vi "UI final scorbot.vi"() -> ()   [LabVIEW 2014]
uses:
  <vilib>/userdefined/High Color/IMAQdx.ctl
  <vilib>/myRIO/Instrument Drivers/Onboard IO/DIO/typedefs/DIO Reference.ctl
  <vilib>/myRIO/Common/Instrument Driver Framework/Utilities/typedefs/myRIO Generic Hardware Reference.ctl
  <vilib>/myRIO/Common/Instrument Driver Framework/Utilities/typedefs/Hardware Version Enum.ctl
  <vilib>/myRIO/Common/Instrument Driver Framework/Utilities/typedefs/myRIO v1.0 Reference.ctl
  <vilib>/myRIO/Common/Instrument Driver Framework/Utilities/typedefs/Generic FPGA Reference.ctl
  <vilib>/myRIO/Common/Instrument Driver Framework/myRIO v1.0/DIO/typedefs/DIO Channels List.ctl
  <vilib>/myRIO/Common/Instrument Driver Framework/myRIO v1.0/DIO/typedefs/DIO Channels Enum.ctl
  <vilib>/userdefined/High Color/nirio_resource_hc.ctl
  <vilib>/myRIO/Common/Instrument Driver Framework/Utilities/vis/Is FPGA Ref Available.vi
  <vilib>/myRIO/Common/Instrument Driver Framework/myRIO v1.0/DIO/vis/myRIO v1.1 Open DIO.vi
  <vilib>/myRIO/Instrument Drivers/Onboard IO/DIO/vis/Read.vi
  <vilib>/myRIO/Common/Instrument Driver Framework/Utilities/vis/Validate Channels.vi
  <vilib>/myRIO/Common/Instrument Driver Framework/myRIO v1.0/DIO/vis/myRIO v1.0 Reserve DIO.vi
  <vilib>/myRIO/Common/Instrument Driver Framework/myRIO v1.0/UART/vis/myRIO v1.0 Close UART.vi
  <vilib>/myRIO/Common/Instrument Driver Framework/myRIO v1.0/Resource Manager/vis/myRIO v1.0 Reserve Channel List.vi
  <vilib>/myRIO/Common/Instrument Driver Framework/myRIO v1.0/DIO/vis/myRIO v1.0 Build MUX Configuration DIO.vi
  <vilib>/myRIO/Common/Instrument Driver Framework/myRIO v1.0/Resource Manager/vis/myRIO v1.0 Reserve Channel.vi
  <vilib>/myRIO/Common/Instrument Driver Framework/myRIO v1.0/Resource Manager/vis/myRIO v1.0 Unreserve Channel.vi
  <vilib>/myRIO/Common/Instrument Driver Framework/myRIO v1.0/Resource Manager/vis/myRIO v1.0 Create Configuration List.vi
  <vilib>/myRIO/Common/Instrument Driver Framework/myRIO v1.0/Resource Manager/vis/myRIO v1.0 Build Mutex Name.vi
  <vilib>/Utility/VariantDataType/GetNumericInfo.vi
  <vilib>/Utility/error.llb/Error Cluster From Error Code.vi
  <vilib>/myRIO/Common/Instrument Driver Framework/myRIO v1.0/myRIO v1.1 Open.vi
  <vilib>/myRIO/Common/Instrument Driver Framework/Utilities/vis/IO Manager.vi
  <vilib>/myRIO/Common/Instrument Driver Framework/Utilities/vis/Configuration Manager.vi
  <vilib>/myRIO/Common/Instrument Driver Framework/myRIO v1.0/Resource Manager/vis/myRIO v1.0 Configure IO.vi
  <vilib>/myRIO/Common/Instrument Driver Framework/myRIO v1.0/myRIO v1.0 Close.vi
  <vilib>/myRIO/Common/Instrument Driver Framework/myRIO v1.0/DIO/vis/myRIO v1.0 Read DIO.vi
  <vilib>/addons/control/pid/pid.llb/PID (DBL).vi
  <vilib>/myRIO/Common/Instrument Driver Framework/Utilities/vis/FPGA Ref Manager.vi
  <vilib>/myRIO/Common/Instrument Driver Framework/myRIO v1.0/myRIO v1.0 Reset FPGA.vi
  <vilib>/myRIO/Common/Instrument Driver Framework/myRIO v1.0/IRQ/vis/myRIO v1.0 IRQ Info FGV.vi
  <vilib>/myRIO/Common/Instrument Driver Framework/myRIO v1.0/IRQ/vis/myRIO v1.0 Timer IRQ Info FGV.vi
  <vilib>/myRIO/Common/Instrument Driver Framework/myRIO v1.0/IRQ/vis/myRIO v1.0 ISR Agent.vi
  <vilib>/Utility/inputDevices.llb/joystickAcquire.vi
  <vilib>/myRIO/Express VI/Onboard IO/DI/DI Express VI.xnode
  <vilib>/myRIO/Instrument Drivers/Onboard IO/DIO/vis/myRIO DIO Open.xnode
  <vilib>/myRIO/Instrument Drivers/Onboard IO/DIO/DIO.lvlib
  <vilib>/addons/control/pid/NI_PID_pid.lvlib
  <vilib>/myRIO/Instrument Drivers/Utilities/Utilities.lvlib
  <vilib>/vision/NI_Vision_Development_Module.lvlib
  <vilib>/vision/driver/NI_Vision_Acquisition_Software.lvlib
panel:
  out "output cluster 5":T1
  out "Numeric 3":dbl
  in  "Reset1":bool
  out "device ID":refnum<k1>
  out "dtheta2":i32
  out "dtheta3":i32
  out "dt":u32
  out "error out 2":errorcluster
  out "output cluster 4":cluster{dbl, dbl}
  out "output cluster 3":cluster{dbl, dbl}
  out "output cluster 2":cluster{dbl, dbl}
  in  "stop VI":bool
  in  "Tab Control":enum32{"Control", "Train"}(tab)
  out "B/DIO3 (Pin 17)":bool
  out "B/DIO2 (Pin 15)":bool
  out "B/DIO4 (Pin 19)":bool
  out "B/DIO5 (Pin 21)":bool
  out "B/DIO6 (Pin 23)":bool
  out "B/DIO7 (Pin 25)":bool
  out "Counter Value 1":dbl
  in  "PID gains 2":T2={"proportional gain (Kc)"=-0.5, "integral time (Ti, min)"=0.0, "derivative time (Td, min)"=0.0} {"derivative time (Td, min)" format="%.3f"; "integral time (Ti, min)" format="%.3f"; "proportional gain (Kc)" format="%.3f"}
  in  "PID gains":T2={"proportional gain (Kc)"=-0.1, "integral time (Ti, min)"=0.0, "derivative time (Td, min)"=0.0} {"derivative time (Td, min)" format="%.3f"; "integral time (Ti, min)" format="%.3f"; "proportional gain (Kc)" format="%.3f"}
  out "Omega3":dbl
  out "Omega2":dbl
  out "Elbow angle":dbl
  in  "Max Angle 3":dbl=90.0
  in  "Min angle 3":dbl=-120.0
  in  "Max Encoder Value 3":dbl=-62000.0
  in  "Min Encoder Value 3":dbl
  out "Shoulder angle":dbl
  in  "Max Angle 2":dbl=120.0
  in  "Min angle 2":dbl
  in  "Max Encoder Value 2":dbl=27000.0
  in  "Min Encoder Value 2":dbl
  out "Base angle":dbl
  in  "Max Angle":dbl=90.0
  in  "Min angle":dbl=-90.0
  in  "Max Encoder Value":dbl=-570.0
  in  "Min Encoder Value":dbl
  in  "Reset":bool
  out "Counter Value 3":i32
  out "Counter Value 2":i32
  out "direction info":T3
  out "button info":T4
  out "axis info":T5
  in  "Tab Control 2":enum32{"Learn", "Perform"}(tab)
  in  "Stop counting":bool
  in  "NEXT":bool
  in  "Tab Control 3":enum32{"Normal training", "Train using Vision"}(tab)=enum."Train using Vision"
  out "Encoders initialised":bool
  in  "Save":bool
  out "output cluster":T6
  in  "Save":bool
  in  "Red or Hue Range":cluster{dbl, dbl}(slide)={0.0, 255.0} scale=0.0..255.0
  out "box area":dbl
  in  "Session In":T7="cam0"
  out "object height":i32
  out "object width":i32
  out "Bottom y-displacement":i32
  out "Right x-displacement":i32
  out "Top y-displacement":i32
  out "Left x-displacement":i32
  out "centroid y-displacement":sgl
  out "centroid x-displacement":sgl
  out "threshold":T8(plugin-control)
  in  "Blue or Luma or Val or Inten Range":cluster{dbl, dbl}(slide)={0.0, 255.0} scale=0.0..255.0
  out "Object Info":T9
  out "Largest Area":sgl
  out "Found Objects":T10(array[cluster]) {"Aspect Ratio" format="%.2f"; "Orientation" format="%.2f"; "Area" format="%.2f"; "Object Center"."Y" format="%.2f"; "Object Center"."X" format="%.2f"}
  out "Number of Objects":i32
  out "live feed":T8(plugin-control)
  in  "Green or Sat Range":cluster{dbl, dbl}(slide)={0.0, 255.0} scale=0.0..255.0
  in  "stop vision":bool
  out "Vision initialised":bool
  out "steps":dbl
  out "Set Elbow":dbl
  out "Set Shoulder":dbl
  out "Set Base":dbl
  in  "NeXT step":dbl
  in  "Max Encoder3":dbl=-118000.0
  in  "Max Encoder 2":dbl=27000.0
  out "data out":dbl[][](array[numeric])
  out "Current Angle 1":dbl
  out "Counter1":dbl
  out "B/DIO3 (Pin 17) 2":bool
  out "B/DIO2 (Pin 15) 2":bool
  out "Set Point1":dbl
  out "direction_1b":bool
  out "direction_1a":bool
  in  "Max Encoder1":dbl=-3300.0
  in  "Reset1":bool
  in  "Set Point Angle1":dbl
  in  "Min Encoder1":dbl
  in  "Min Angle1":dbl=-90.0
  in  "Max Angle1":dbl=90.0
  out "error 3":dbl
  in  "Enable1":bool=TRUE
  out "Current Angle3":dbl
  out "direction_3b":bool
  out "B/DIO6 (Pin 23) 2":bool
  out "B/DIO7 (Pin 25) 2":bool
  out "dirction_3a":bool
  out "Set Point3":dbl
  in  "Reset3":bool
  in  "Set Point Angle3":dbl
  out "Numeric3":dbl
  out "Omega3 2":dbl
  out "dt 2":u32
  out "dtheta":i32
  in  "Min Encoder3":dbl
  in  "Min Angle3":dbl=-120.0
  in  "Max Angle3":dbl=90.0
  out "error3":dbl
  out "Counter Value3":i32
  out "B/DIO5 (Pin 21) 2":bool
  out "B/DIO4 (Pin 19) 2":bool
  out "direction 2b":bool
  out "direction 2a":bool
  out "Current Angle2":dbl
  in  "Reset 2":bool
  in  "Set Point Angle2":dbl
  out "Numeric2":dbl
  out "Omega 2":dbl
  out "dt 3":u32
  out "dtheta 2":i32
  in  "PID gains 4":T2={"proportional gain (Kc)"=-0.5, "integral time (Ti, min)"=0.0, "derivative time (Td, min)"=0.0} {"derivative time (Td, min)" format="%.3f"; "integral time (Ti, min)" format="%.3f"; "proportional gain (Kc)" format="%.3f"}
  in  "Min Encoder2":dbl
  in  "Min Angle2":dbl
  in  "Max Angle2":dbl=120.0
  out "error 2":dbl
  in  "Set Point2":dbl
  out "Counter Value2":i32
  in  "PID gains 3":T2={"proportional gain (Kc)"=-0.1, "integral time (Ti, min)"=0.0, "derivative time (Td, min)"=0.0} {"derivative time (Td, min)" format="%.3f"; "integral time (Ti, min)" format="%.3f"; "proportional gain (Kc)" format="%.3f"}
  out "Array":dbl[][](array[numeric])
  out "Array 2":dbl[][](array[numeric])
  out "Array 3":dbl[][](array[numeric])
  out "Array 4":dbl[][](array[numeric])
  out "Array 5":dbl[][](array[numeric])
  out "Array 6":dbl[][](array[numeric])
types:
  T1 = cluster{dbl[][], dbl[][], dbl[][], dbl[][], dbl[][], dbl[][]}
  T2 = cluster{"proportional gain (Kc)":dbl, "integral time (Ti, min)":dbl, "derivative time (Td, min)":dbl}
  T3 = cluster{"pov 1":i32, "pov 2":i32, "pov 3":i32, "pov 4":i32}
  T4 = cluster{"button 1":bool, "button 2":bool, "button 3":bool, "button 4":bool, "button 5":bool, "button 6":bool, "button 7":bool, "button 8":bool, "button 9":bool, "button 10":bool, "button 11":bool, "button 12":bool, "button 13":bool, "button 14":bool, "button 15":bool, "button 16":bool, "button 17":bool, "button 18":bool, "button 19":bool, "button 20":bool, "button 21":bool, "button 22":bool, "button 23":bool, "button 24":bool, "button 25":bool, "button 26":bool, "button 27":bool, "button 28":bool, "button 29":bool, "button 30":bool, "button 31":bool, "button 32":bool}
  T5 = cluster{"X axis":i32, "Y axis":i32, "Z axis":i32, "X axis rotation":i32, "Y axis rotation":i32, "Z axis rotation":i32, "U axis":i32, "V axis":i32}
  T6 = cluster{"Elbow angle":dbl, "Base angle":dbl, "Shoulder angle":dbl}
  T7 = typedef "IMAQdx.ctl" = refnum<k21>
  T8 = typedef "IMAQ Image.ctl" = refnum<image>
  T9 = cluster{"Object Center":cluster{"X":sgl, "Y":sgl}, "Bounding Box":cluster{"X Left":i32, "Y Top":i32, "X Right":i32, "Y Bottom":i32}, "Area":sgl, "Orientation":sgl, "Aspect Ratio":sgl, "Nb Holes":i32}
  T10 = cluster{"Object Center":cluster{"X":sgl, "Y":sgl}, "Bounding Box":cluster{"X Left":i32, "Y Top":i32, "X Right":i32, "Y Bottom":i32}, "Area":sgl, "Orientation":sgl, "Aspect Ratio":sgl, "Nb Holes":i32}[]
  T11 = cluster{"Objects":u16, "Threshold":i32, "Reject Border":bool, "Fill Holes":bool, "Min Object Size":bool, "Min Size":i32, "Max Object Size":bool, "Max Size":i32, "Show Search Area":bool, "Show Center":bool, "Show Bounding Box":bool}
  T12 = typedef "DIO.lvlib/DIO Reference.ctl" = cluster{"myRIO Reference":T13, "DIO Channels List":T17}
  T13 = typedef "myRIO Generic Hardware Reference.ctl" = cluster{"myRIO Model":T14, "myRIO Hardware Reference":T15}
  T14 = typedef "Hardware Version Enum.ctl" = enum16{"Unknown", "myRIO-1900", "myRIO-1950"}
  T15 = typedef "myRIO v1.0 Reference.ctl" = cluster{"Generic FPGA Reference":T16, "Allow multiple opens":bool}
  T16 = typedef "Generic FPGA Reference.ctl" = refnum<k20>
  T17 = typedef "DIO Channels List.ctl" = T18[]
  T18 = typedef "DIO Channels Enum.ctl" = enum16{"Not Connected", "C/DIO0", "C/DIO1", "C/DIO2", "C/DIO3", "C/DIO4", "C/DIO5", "C/DIO6", "C/DIO7", "A/DIO0", "A/DIO1", "A/DIO2", "A/DIO3", "A/DIO4", "A/DIO5", "A/DIO6", "A/DIO7", "A/DIO8", "A/DIO9", "A/DIO10", "A/DIO11", "A/DIO12", "A/DIO13", "A/DIO14", "A/DIO15", "B/DIO0", "B/DIO1", "B/DIO2", "B/DIO3", "B/DIO4", "B/DIO5", "B/DIO6", "B/DIO7", "B/DIO8", "B/DIO9", "B/DIO10", "B/DIO11", "B/DIO12", "B/DIO13", "B/DIO14", "B/DIO15", "LED0", "LED1", "LED2", "LED3", "Button0"}
  T19 = typedef "nirio_resource_hc.ctl" = tag
  T20 = typedef "Image Type" = u32
  T21 = cluster{"X Left":i32, "Y Top":i32, "X Right":i32, "Y Bottom":i32}
  T22 = typedef "NI_Matrix.lvlib/RealMatrix.ctl" = dbl[][]
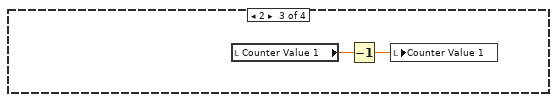
[diagram p8: hidden frame]
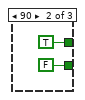
[diagram p10: hidden frame]
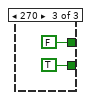
[diagram p11: hidden frame]
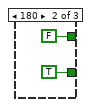
[diagram p12: hidden frame]
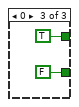
[diagram p13: hidden frame]
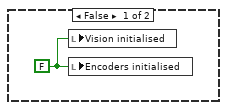
[diagram p16: hidden frame]
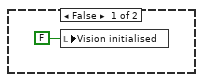
[diagram p17: hidden frame]
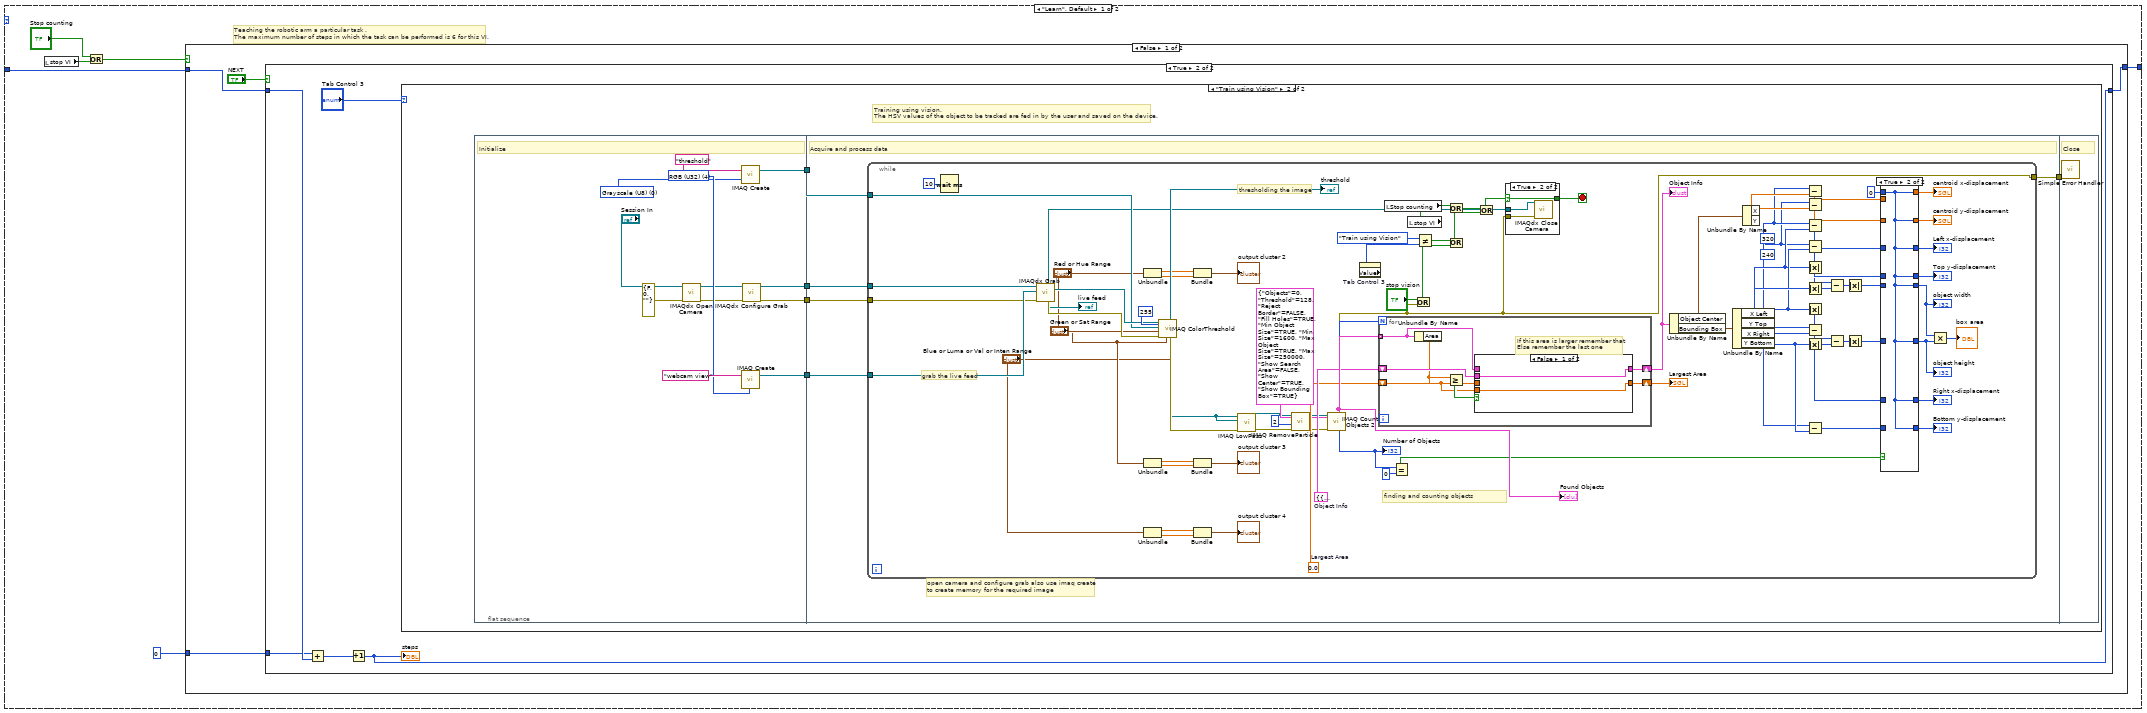
[diagram p19: hidden frame]
diagram:
  # "You can configure the Accelerometer Express VI by double-clicking it.\nYou can find other myRIO Express VIs in the myRIO palette."
  n1 = flat-sequence {
    tunnel: [errorcluster {"status"=FALSE, "code"=0, "source"=""} ("error out")] -> w3
    tunnel: [w4] -> w2
    tunnel: w3 -> [w9]
    tunnel: w2 -> [w10]
    tunnel: [w6] -> w1
    tunnel: w1 -> [w799]
    frame #0 {
      # "train1"
      # "#CodeNeeded - Add code to initialize your user interface and hardware here."
      # "Initialize"
      n2 = call <vilib>:"Initialize Joystick.vi"() -> ("device ID"=w4:refnum<k1>)  [unwired: 10 in, 1 out]
      "device ID" <- w4
    }
    frame #1 {
      # "Network Stream:\nFile Reader and Writer"
      # "train1"
      # "n3"
      # "n2"
      # "n1"
      # "host VI"
      # "Acquire and process data"
      n3 = while {
        shift-right: [w137] -> _
        shift-left: _ -> [w136]
        tunnel: w10 -> [w121]
        stop <- "stop VI" stop-if-true
        # "Network streams are used to transfer the encoder and \nvision data from myRio to the computer and vice versa."
        # "n3"
        # "n2"
        # "n1"
        n4 = local read "Tab Control 2"() -> (w134:enum32{"Learn", "Perform"})
        n5 = local read "Tab Control"() -> (w132:enum32{"Control", "Train"})
        n6 = case shown="\"Train\"" "Tab Control" {
          tunnel: [w149 w152] -> w137
          tunnel: w136 -> [w149 w151]
          tunnel: w121 -> [_ _]
          frame "Control", Default {
          }
          frame "Train" {
            # "Training the robotic arm by moving it using joystick.\nThe initial and final encoder readings of each arm are \nbeing transferred to the computer in each step."
            n7 = case shown="\"Perform\"" "Tab Control 2" {
              tunnel: [w158 w302] -> w152
              tunnel: w151 -> [w156 w302]
              frame "Learn", Default {
                # "Teaching the robotic arm a particular task .\nThe maximum number of steps in which the task can be performed is 6 for this VI."
                n8 = local read "stop VI"() -> (w154:bool)
                n9 = Or(x="Stop counting", y=w154) -> (x .or. y?=w153:bool)
                n10 = case shown="False" w153 {
                  tunnel: [w162 w301] -> w158
                  tunnel: 0 -> [w160 w299]
                  tunnel: w156 -> [w159 w300]
                  frame False {
                    n11 = case shown="True" "NEXT" {
                      tunnel: [w163 w165] -> w162
                      tunnel: w159 -> [w163 w167]
                      tunnel: w160 -> [_ w166]
                      frame False {
                      }
                      frame True {
                        n12 = Add(x=w166, y=w167) -> (x+y=w168:i32)
                        n13 = Increment(x=w168) -> (x+1=w165:i32)
                        "steps" <- w165
                        n14 = case shown="\"Train using Vision\"" "Tab Control 3" {
                          frame "Normal training", Default {
                            # "Training by storing encoder readings"
                          }
                          frame "Train using Vision" {
                            # "Training using vision. \nThe HSV values of the object to be tracked are fed in by the user and saved on the device."
                            n15 = flat-sequence {
                              tunnel: [w183] -> w173
                              tunnel: [w180] -> w172
                              tunnel: [w177] -> w171
                              tunnel: [w174] -> w170
                              tunnel: w173 -> [w189]
                              tunnel: [w186] -> w169
                              tunnel: w172 -> [w188]
                              tunnel: w171 -> [w187]
                              tunnel: w170 -> [w190]
                              tunnel: w169 -> [w298]
                              frame #0 {
                                w175 = T20 0 items=["Grayscale (U8)", "Grayscale (I16)", "Grayscale (SGL)", "Complex (CSG)", "RGB (U32)", "HSL (U32)", "RGB (U64)", "Grayscale (U16)"] ("Image Type")
                                w184 = T20 4 items=["Grayscale (U8)", "Grayscale (I16)", "Grayscale (SGL)", "Complex (CSG)", "RGB (U32)", "HSL (U32)", "RGB (U64)", "Grayscale (U16)"] ("Image Type")
                                # "Initialize"
                                n16 = call <vilib>:"IMAQdx Open Camera.vi"("error in"=errorcluster {"status"=FALSE, "code"=0, "source"=""} ("error out"), "Session In"="Session In") -> ("error out"=w179:errorcluster, "Session Out"=w181:T7)  [unwired: 8 in]
                                n17 = call "IMAQ Create"("Image Name"="threshold", "Image Type"=w175) -> ("New Image"=w174:T8)  [unwired: 3 in, 1 out]
                                n18 = call "IMAQ Create"("Image Name"="webcam view", "Image Type"=w184) -> ("New Image"=w183:T8)  [unwired: 3 in, 1 out]
                                n19 = call <vilib>:"IMAQdx Configure Grab.vi"("error in"=w179, "Session In"=w181) -> ("error out"=w177:errorcluster, "Session Out"=w180:T7)  [unwired: 8 in]
                              }
                              frame #1 {
                                # "open camera and configure grab also use imaq create \nto create memory for the required image"
                                # "Acquire and process data"
                                n20 = while {
                                tunnel: w190 -> [w225]
                                tunnel: w189 -> [w224]
                                tunnel: w188 -> [w215]
                                tunnel: w187 -> [w223]
                                tunnel: [w213] -> w186
                                stop <- w216 stop-if-true
                                w230 = 240
                                w232 = 320
                                w269 = T9 {"Object Center"={"X"=0.0, "Y"=0.0}, "Bounding Box"={"X Left"=0, "Y Top"=0, "X Right"=0, "Y Bottom"=0}, "Area"=0.0, "Orientation"=0.0, "Aspect Ratio"=0.0, "Nb Holes"=0}  # Object Info
                                w268 = sgl 0.0  # Largest Area
                                # "finding and counting objects"
                                # "thresholding the image"
                                # "grab the live feed"
                                n21 = Wait (ms)(milliseconds to wait=u32 10) -> ()  [unwired: 1 out]
                                n22 = call <vilib>:"IMAQdx Grab.vi"("error in"=w223, "Image In"=w224, "Session In"=w215) -> ("error out"=w273:errorcluster, "Image Out"=w271:T8, "Session Out"=w214:T7)  [unwired: 5 in, 1 out]
                                "live feed" <- w271
                                n23 = Unbundle("Red or Hue Range") -> (w199:dbl, w198:dbl)
                                n24 = Unbundle("Green or Sat Range") -> (w197:dbl, w196:dbl)
                                n25 = Unbundle("Blue or Luma or Val or Inten Range") -> (w195:dbl, w194:dbl)
                                n26 = call "IMAQ ColorThreshold"("Blue or Luma or Val or Inten Range"="Blue or Luma or Val or Inten Range", "Replace Value"=255, "Green or Sat Range"="Green or Sat Range", "error in (no error)"=w273, "Red or Hue Range"="Red or Hue Range", "Image Dst"=w225, "Image Src"=w271) -> ("error out"=w266:errorcluster, "Image Dst Out"=w265:T8)  [unwired: 3 in]
                                "threshold" <- w265
                                n27 = Bundle(w199, w198) -> (→"output cluster 2":cluster{dbl, dbl})  [unwired: 1 in]
                                n28 = Bundle(w197, w196) -> (→"output cluster 3":cluster{dbl, dbl})  [unwired: 1 in]
                                n29 = Bundle(w195, w194) -> (→"output cluster 4":cluster{dbl, dbl})  [unwired: 1 in]
                                n30 = call "IMAQ LowPass"("Image Src"=w265, "Image Mask"=w265, "error in (no error)"=w266) -> ("Image Dst Out"=w227:T8, "error out"=w229:errorcluster)  [unwired: 4 in]
                                n31 = call "IMAQ RemoveParticle"("error in (no error)"=w229, "Number of Erosion"=2, "Image Src"=w227) -> ("error out"=w228:errorcluster, "Image Dst Out"=w226:T8)  [unwired: 7 in]
                                n32 = call "IMAQ Count Objects 2"("Settings"=T11 {"Objects"=0, "Threshold"=128, "Reject Border"=FALSE, "Fill Holes"=TRUE, "Min Object Size"=TRUE, "Min Size"=1600, "Max Object Size"=TRUE, "Max Size"=250000, "Show Search Area"=FALSE, "Show Center"=TRUE, "Show Bounding Box"=TRUE}, "error in (no error)"=w228, "Image"=w226) -> ("error out"=w213:errorcluster, "Number of Objects"=w259:i32, "Objects"=w270:T10)  [unwired: 4 in, 2 out]
                                "Number of Objects" <- w259
                                "Found Objects" <- w270
                                n33 = property on="Tab Control 3" class="TabCtl (strict)"() -> ("Value"=w210:enum32{"Normal training", "Train using Vision"})  [unwired: 2 in, 2 out]
                                n34 = for {
                                N: w259 -> [_]
                                tunnel: w270 -> [w290] mode=indexing
                                shift-right: [w293] -> w267
                                shift-left: w268 -> [w287]
                                shift-right: [w292] -> w264
                                shift-left: w269 -> [w291]
                                # "If this area is larger remember that\nElse remember the last one"
                                n35 = Unbundle By Name(w290) -> ("Area"=w289:sgl)
                                n36 = Greater Or Equal?(x=w289, y=w287) -> (x >= y?=w288:bool)
                                n37 = case shown="False" w288 {
                                tunnel: [w295 w297] -> w293
                                tunnel: w289 -> [_ w297]
                                tunnel: w287 -> [w295 _]
                                tunnel: [w294 w296] -> w292
                                tunnel: w291 -> [w294 _]
                                tunnel: w290 -> [_ w296]
                                frame False {
                                }
                                frame True {
                                }
                                }
                                }
                                "Largest Area" <- w267
                                "Object Info" <- w264
                                n38 = local read "Stop counting"() -> (w207:bool)
                                n39 = Equal?(x=w259, y=0) -> (x = y?=w257:bool)
                                n40 = local read "stop VI"() -> (w206:bool)
                                n41 = Or(x="stop vision", y=w213) -> (x .or. y?=w211:bool)
                                n42 = Not Equal?(x=enum32{"Normal training", "Train using Vision"}."Train using Vision" ("Tab Control 3"), y=w210) -> (x != y?=w212:bool)
                                n43 = Or(x=w207, y=w206) -> (x .or. y?=w205:bool)
                                n44 = Or(x=w212, y=w211) -> (x .or. y?=w204:bool)
                                n45 = Or(x=w205, y=w204) -> (x .or. y?=w203:bool)
                                n46 = case shown="True" w203 {
                                selector: w203 -> [_ w276]
                                tunnel: w213 -> [_ w275]
                                tunnel: [FALSE w276] -> w216
                                tunnel: w214 -> [_ w277]
                                frame False {
                                }
                                frame True {
                                n47 = call <vilib>:"IMAQdx Close Camera.vi"("error in"=w275, "Session In"=w277) -> ()  [unwired: 9 in, 1 out]
                                }
                                }
                                n48 = Unbundle By Name(w264) -> ("Object Center"=w263:cluster{"X":sgl, "Y":sgl}, "Bounding Box"=w261:T21)
                                n49 = Unbundle By Name(w261) -> ("X Left"=w233:i32, "Y Top"=w234:i32, "X Right"=w235:i32, "Y Bottom"=w231:i32)
                                n50 = Unbundle By Name(w263) -> ("X"=w237:sgl, "Y"=w236:sgl)
                                n51 = Subtract(x=w232, y=w237) -> (x-y=w251:sgl)
                                n52 = Subtract(x=w230, y=w236) -> (x-y=w250:sgl)
                                n53 = Subtract(x=w232, y=w233) -> (x-y=w249:i32)
                                n54 = Subtract(x=w230, y=w234) -> (x-y=w248:i32)
                                n55 = Absolute Value(x=w233) -> (abs(x)=w243:i32)
                                n56 = Absolute Value(x=w235) -> (abs(x)=w242:i32)
                                n57 = Absolute Value(x=w234) -> (abs(x)=w245:i32)
                                n58 = Subtract(x=w232, y=w235) -> (x-y=w247:i32)
                                n59 = Absolute Value(x=w231) -> (abs(x)=w244:i32)
                                n60 = Subtract(x=w230, y=w231) -> (x-y=w246:i32)
                                n61 = Subtract(x=w243, y=w242) -> (x-y=w241:i32)
                                n62 = Subtract(x=w245, y=w244) -> (x-y=w239:i32)
                                n63 = Absolute Value(x=w241) -> (abs(x)=w240:i32)
                                n64 = Absolute Value(x=w239) -> (abs(x)=w238:i32)
                                n65 = case shown="True" w257 {
                                tunnel: [w285 w286] -> w222
                                tunnel: 0 -> [_ w286]
                                tunnel: [w284 w286] -> w221
                                tunnel: [w283 w286] -> w255
                                tunnel: [w281 w286] -> w254
                                tunnel: [w282 w286] -> w253
                                tunnel: [w280 w286] -> w252
                                tunnel: w251 -> [w285 _]
                                tunnel: w250 -> [w284 _]
                                tunnel: w249 -> [w283 _]
                                tunnel: w248 -> [w282 _]
                                tunnel: w247 -> [w281 _]
                                tunnel: w246 -> [w280 _]
                                tunnel: [w279 w286] -> w219
                                tunnel: w240 -> [w279 _]
                                tunnel: [w278 w286] -> w218
                                tunnel: w238 -> [w278 _]
                                frame False {
                                }
                                frame True {
                                }
                                }
                                "centroid x-displacement" <- w222
                                "centroid y-displacement" <- w221
                                "Left x-displacement" <- w255
                                "Top y-displacement" <- w253
                                "Right x-displacement" <- w254
                                "Bottom y-displacement" <- w252
                                "object width" <- w219
                                "object height" <- w218
                                n66 = Multiply(x=w219, y=w218) -> (x*y=→"box area":i32)
                                }
                              }
                              frame #2 {
                                # "Close"
                                n67 = call <vilib>:"Simple Error Handler.vi"("error in (no error)"=w298) -> ()  [unwired: 4 in, 5 out]
                              }
                            }
                          }
                        }
                      }
                    }
                  }
                  frame True {
                    n68 = Multiply(x=w299, y=w300) -> (x*y=w301:i32)
                  }
                }
              }
              frame "Perform" {
                # "The Robotic arm performs the task autonomously in steps.\nThe myRio reads the initial and final encoder readings from the file on \ncomputer and actuates the motors accordingly to reach the desired position."
                n69 = while {
                  tunnel: [w366] -> _
                  shift-right: [w482] -> _
                  shift-left: _ -> [w483]
                  shift-right: [w479] -> _
                  shift-left: _ -> [w481]
                  shift-right: [w478] -> _
                  shift-left: _ -> [w480]
                  shift-right: [w421] -> _
                  shift-left: _ -> [w424]
                  shift-right: [w420] -> _
                  shift-left: _ -> [w423]
                  shift-right: [w419] -> _
                  shift-left: _ -> [w422]
                  shift-right: [w364] -> _
                  shift-left: _ -> [w365]
                  stop <- w304 stop-if-true
                  # "PID for speed control"
                  # "PID for speed control"
                  n70 = local read "output cluster 5"() -> (w315:T1)
                  n71 = local read "Tab Control 2"() -> (w307:enum32{"Learn", "Perform"})
                  n72 = local read "Set Shoulder"() -> (w310:dbl)
                  n73 = local read "Set Point1"() -> (w346:dbl)
                  n74 = local read "Set Elbow"() -> (w309:dbl)
                  n75 = local read "Counter1"() -> (w336:dbl)
                  n76 = local read "Set Base"() -> (w308:dbl)
                  n77 = local write "Set Point Angle2"(w310) -> ()
                  n78 = local write "Set Point Angle1"(w308) -> ()
                  n79 = case shown="True" "Reset1" {
                    frame False {
                    }
                    frame True {
                      n80 = local write "Counter1"(0.0 ("Counter")) -> ()
                    }
                  }
                  n81 = local write "Set Point Angle3"(w309) -> ()
                  n82 = case shown="0, Default" "NeXT step" {
                    tunnel: w315 -> [_ w492 w505 w514 w523 w531 w541]
                    tunnel: [w491 w499 w503 w512 w521 w530 w539] -> w313
                    tunnel: [w490 w495 w502 w511 w520 w529 w538] -> w312
                    tunnel: [w489 w494 w501 w510 w519 w528 w537] -> w311
                    frame 0, Default {
                      n83 = local read "Current Angle 1"() -> (w490:dbl)
                      n84 = local read "Current Angle3"() -> (w491:dbl)
                      n85 = local read "Current Angle2"() -> (w489:dbl)
                    }
                    frame 1 {
                      w496 = 0 ("index (col)")
                      n86 = Unbundle(w492) -> (w493:dbl[][])  [unwired: 5 out]
                      n87 = Index Array(array=w493, index (row) #1=0 ("index (row)"), index (col) #1=w496, index (row) #2=1 ("index (row)"), index (col) #2=w496, index (row) #3=2 ("index (row)"), index (col) #3=w496) -> (element #1=w499:dbl, element #2=w495:dbl, element #3=w494:dbl)
                    }
                    frame 2 {
                      w506 = 0 ("index (col)")
                      n88 = Unbundle(w505) -> (w504:dbl[][])  [unwired: 5 out]
                      n89 = Index Array(array=w504, index (row) #1=0 ("index (row)"), index (col) #1=w506, index (row) #2=1 ("index (row)"), index (col) #2=w506, index (row) #3=2 ("index (row)"), index (col) #3=w506) -> (element #1=w503:dbl, element #2=w502:dbl, element #3=w501:dbl)
                    }
                    frame 3 {
                      w515 = 0 ("index (col)")
                      n90 = Unbundle(w514) -> (w513:dbl[][])  [unwired: 5 out]
                      n91 = Index Array(array=w513, index (row) #1=0 ("index (row)"), index (col) #1=w515, index (row) #2=1 ("index (row)"), index (col) #2=w515, index (row) #3=2 ("index (row)"), index (col) #3=w515) -> (element #1=w512:dbl, element #2=w511:dbl, element #3=w510:dbl)
                    }
                    frame 4 {
                      w524 = 0 ("index (col)")
                      n92 = Unbundle(w523) -> (w522:dbl[][])  [unwired: 5 out]
                      n93 = Index Array(array=w522, index (row) #1=0 ("index (row)"), index (col) #1=w524, index (row) #2=1 ("index (row)"), index (col) #2=w524, index (row) #3=2 ("index (row)"), index (col) #3=w524) -> (element #1=w521:dbl, element #2=w520:dbl, element #3=w519:dbl)
                    }
                    frame 5 {
                      w536 = 0 ("index (col)")
                      n94 = Unbundle(w531) -> (w532:dbl[][])  [unwired: 5 out]
                      n95 = Index Array(array=w532, index (row) #1=0 ("index (row)"), index (col) #1=w536, index (row) #2=1 ("index (row)"), index (col) #2=w536, index (row) #3=2 ("index (row)"), index (col) #3=w536) -> (element #1=w530:dbl, element #2=w529:dbl, element #3=w528:dbl)
                    }
                    frame 6 {
                      w542 = 0 ("index (col)")
                      n96 = Unbundle(w541) -> (w540:dbl[][])  [unwired: 5 out]
                      n97 = Index Array(array=w540, index (row) #1=0 ("index (row)"), index (col) #1=w542, index (row) #2=1 ("index (row)"), index (col) #2=w542, index (row) #3=2 ("index (row)"), index (col) #3=w542) -> (element #1=w539:dbl, element #2=w538:dbl, element #3=w537:dbl)
                    }
                  }
                  "Set Elbow" <- w313
                  "Set Base" <- w312
                  "Set Shoulder" <- w311
                  n98 = Not Equal?(x=w307, y=enum32{"Learn", "Perform"}."Perform" ("Tab Control 2")) -> (x != y?=w305:bool)
                  n99 = local read "Numeric 3"() -> (w358:dbl)
                  n100 = local read "Numeric 3"() -> (w356:dbl)
                  n101 = Subtract(x=w336, y=w346) -> (x-y=w361:dbl)
                  "error 3" <- w361
                  n102 = Subtract(x="Max Angle1", y="Min Angle1") -> (x-y=w322:dbl)
                  n103 = Subtract(x="Max Encoder1", y="Min Encoder1") -> (x-y=w321:dbl)
                  n104 = local read "stop VI"() -> (w303:bool)
                  n105 = Subtract(x="Set Point Angle1", y="Min Angle1") -> (x-y=w350:dbl)
                  n106 = Divide(x=w321, y=w322) -> (x/y=w349:dbl)
                  n107 = Divide(x=w322, y=w321) -> (x/y=w320:dbl)
                  n108 = Add(x=1.0 ("upper limit"), y=w358) -> (x+y=w359:dbl)
                  n109 = Subtract(x=-1.0 ("lower limit"), y=w356) -> (x-y=w355:dbl)
                  n110 = xnode "Digital input (1 sample) 7"() -> ("B/DIO6 (Pin 23)"=w384:bool)  [unwired: 1 in, 1 out]
                  "B/DIO6 (Pin 23) 2" <- w384
                  n111 = Or(x=w305, y=w303) -> (x .or. y?=w304:bool)
                  n112 = Multiply(x=w350, y=w349) -> (x*y=w348:dbl)
                  n113 = local read "Counter1"() -> (w319:dbl)
                  n114 = In Range and Coerce(upper limit=w359, x=w361, lower limit=w355) -> (In Range?=w345:bool)  [unwired: 1 out]
                  n115 = Sign(1:w361) -> (0:w363:dbl)
                  n116 = xnode "Digital input (1 sample) 8"() -> ("B/DIO7 (Pin 25)"=w382:bool)  [unwired: 1 in, 1 out]
                  "B/DIO7 (Pin 25) 2" <- w382
                  n117 = case shown="True" w345 {
                    frame False {
                      n118 = local write "Numeric 3"(0.0) -> ()
                    }
                    frame True {
                      n119 = local write "Numeric 3"(0.0) -> ()
                    }
                  }
                  n120 = case shown="1" w363 {
                    tunnel: [TRUE TRUE FALSE] -> w342
                    tunnel: [TRUE FALSE TRUE] -> w343
                    frame 0, Default {
                    }
                    frame 1 {
                    }
                    frame -1 {
                    }
                  }
                  n121 = Add(x=w348, y="Min Encoder1") -> (x+y=w340:dbl)
                  n122 = Multiply(x=w320, y=w319) -> (x*y=w318:dbl)
                  n123 = local write "Set Point1"(w340) -> ()
                  n124 = Add(x="Min Angle1", y=w318) -> (x+y=→"Current Angle 1":dbl)
                  n125 = feedback #1() -> (w385:bool)  [unwired: 1 in]
                  n126 = Not(x=w384) -> (.not. x?=w387:bool)
                  n127 = And(x=w385, y=w382) -> (x .and. y?=w383:bool)
                  "dirction_3a" <- w383
                  n128 = Not(x=w345) -> (.not. x?=w344:bool)
                  n129 = Or(x=w387, y="Reset3") -> (x .or. y?=w394:bool)
                  n130 = And(x=w344, y=w342) -> (x .and. y?=w335:bool)
                  n131 = And(x=w344, y=w343) -> (x .and. y?=w334:bool)
                  n132 = xnode "Digital input (1 sample) 9"() -> ("B/DIO4 (Pin 19)"=w431:bool)  [unwired: 1 in, 1 out]
                  "B/DIO4 (Pin 19) 2" <- w431
                  n133 = case shown="True" "Enable1" {
                    tunnel: w335 -> [_ w627]
                    tunnel: w334 -> [_ w626]
                    tunnel: [FALSE w627] -> w333
                    tunnel: [FALSE w626] -> w323
                    frame False {
                    }
                    frame True {
                    }
                  }
                  n134 = local read "Set Point3"() -> (w395:dbl)
                  n135 = feedback #2() -> (w368:dbl)  [unwired: 1 in]
                  n136 = Subtract(x="Max Encoder3", y="Min Encoder3") -> (x-y=w377:dbl)
                  n137 = Subtract(x="Max Angle3", y="Min Angle3") -> (x-y=w378:dbl)
                  n138 = Tick Count (ms)() -> (millisecond timer value=w419:u32)
                  n139 = xnode "Digital input (1 sample) 12"() -> ("B/DIO2 (Pin 15)"=w337:bool)  [unwired: 1 in, 1 out]
                  "B/DIO2 (Pin 15) 2" <- w337
                  n140 = Divide(x=w378, y=w377) -> (x/y=w373:dbl)
                  n141 = Divide(x=w377, y=w378) -> (x/y=w398:dbl)
                  n142 = Subtract(x="Set Point Angle3", y="Min Angle3") -> (x-y=w399:dbl)
                  n143 = local read "Numeric3"() -> (w406:dbl)
                  n144 = local read "Numeric3"() -> (w404:dbl)
                  n145 = Not(x=w431) -> (.not. x?=w432:bool)
                  n146 = Subtract(x=w419, y=w422) -> (x-y=w410:u32)
                  "dt 2" <- w410
                  n147 = feedback #3() -> (w448:bool)  [unwired: 1 in]
                  n148 = Multiply(x=w399, y=w398) -> (x*y=w397:dbl)
                  n149 = And(x=w448, y=w431) -> (x .and. y?=w427:bool)
                  "direction 2a" <- w427
                  n150 = Add(x=50.0 ("upper limit"), y=w406) -> (x+y=w407:dbl)
                  n151 = Subtract(x=-50.0 ("lower limit"), y=w404) -> (x-y=w403:dbl)
                  n152 = Or(x=w432, y="Reset 2") -> (x .or. y?=w434:bool)
                  n153 = Add(x=w397, y="Min Encoder3") -> (x+y=w396:dbl)
                  n154 = And(x=w333, y=w337) -> (x .and. y?=w324:bool)
                  "direction_1a" <- w324
                  n155 = local write "Set Point3"(w396) -> ()
                  n156 = Subtract(x="Max Encoder 2", y="Min Encoder2") -> (x-y=w446:dbl)
                  n157 = Subtract(x="Max Angle2", y="Min Angle2") -> (x-y=w447:dbl)
                  n158 = xnode "Digital input (1 sample) 11"() -> ("B/DIO3 (Pin 17)"=w330:bool)  [unwired: 1 in, 1 out]
                  "B/DIO3 (Pin 17) 2" <- w330
                  n159 = local read "Set Point2"() -> (w442:dbl)
                  n160 = Divide(x=w446, y=w447) -> (x/y=w438:dbl)
                  n161 = Divide(x=w447, y=w446) -> (x/y=w445:dbl)
                  n162 = Subtract(x="Set Point Angle2", y="Min Angle2") -> (x-y=w439:dbl)
                  n163 = Boolean To (0,1)(Boolean=w324) -> (0, 1=w329:i16)
                  n164 = Tick Count (ms)() -> (millisecond timer value=w478:u32)
                  n165 = Multiply(x=w439, y=w438) -> (x*y=w437:dbl)
                  n166 = local read "Numeric2"() -> (w454:dbl)
                  n167 = local read "Numeric2"() -> (w452:dbl)
                  n168 = Boolean To (0,1)(Boolean=w323) -> (0, 1=w326:i16)
                  n169 = Subtract(x=w478, y=w480) -> (x-y=w460:u32)
                  "dt 3" <- w460
                  n170 = Multiply(x=i16 2, y=w329) -> (x*y=w327:i16)
                  n171 = Add(x=w327, y=w326) -> (x+y=w325:i16)
                  n172 = Add(x=w437, y="Min Encoder2") -> (x+y=w435:dbl)
                  n173 = And(x=w330, y=w323) -> (x .and. y?=w331:bool)
                  "direction_1b" <- w331
                  n174 = Not(x=w330) -> (.not. x?=w341:bool)
                  n175 = Add(x=50.0 ("upper limit"), y=w454) -> (x+y=w455:dbl)
                  n176 = Subtract(x=-50.0 ("lower limit"), y=w452) -> (x-y=w451:dbl)
                  n177 = case shown="1" w325 {
                    frame 0, Default {
                    }
                    frame 1 {
                      n178 = local read "Counter1"() -> (w547:dbl)
                      n179 = Increment(x=w547) -> (x+1=w546:dbl)
                      n180 = local write "Counter1"(w546) -> ()
                    }
                    frame 2 {
                      n181 = local read "Counter1"() -> (w549:dbl)
                      n182 = Decrement(x=w549) -> (x-1=w548:dbl)
                      n183 = local write "Counter1"(w548) -> ()
                    }
                    frame 3 {
                    }
                  }
                  n184 = local write "Set Point2"(w435) -> ()
                  n185 = Or(x=w341, y="Reset1") -> (x .or. y?=w332:bool)
                  n186 = feedback #4() -> (w433:dbl)  [unwired: 1 in]
                  n187 = case shown="True" w332 {
                    frame False {
                    }
                    frame True {
                      n188 = local write "Counter1"(0.0 ("Counter")) -> ()
                    }
                  }
                  n189 = xnode "Digital input (1 sample) 10"() -> ("B/DIO5 (Pin 21)"=w429:bool)  [unwired: 1 in, 1 out]
                  "B/DIO5 (Pin 21) 2" <- w429
                  n190 = feedback #5() -> (w474:bool)  [unwired: 1 in]
                  n191 = feedback #6() -> (w473:bool)  [unwired: 1 in]
                  n192 = case shown="True" TRUE {
                    tunnel: [FALSE w791] -> w472
                    tunnel: w474 -> [_ w791]
                    tunnel: w473 -> [_ w790]
                    tunnel: [FALSE w790] -> w470
                    frame False {
                    }
                    frame True {
                    }
                  }
                  n193 = feedback #7() -> (w430:bool)  [unwired: 1 in]
                  n194 = local read "output cluster 5"() -> (w488:T1)
                  n195 = And(x=w430, y=w429) -> (x .and. y?=w428:bool)
                  "direction 2b" <- w428
                  n196 = call "SubMotor02.vi"("Reset Counter"=w434, "error in (no error)"=w483, "Duty Cycle"=w433, "A/DIO4 (Pin 19)"=w428, "A/DIO3 (Pin 17)"=w427) -> ("error out"=w482:errorcluster, "Counter Value"=w479:i32)  [unwired: 4 in, 1 out]
                  "Counter Value2" <- w479
                  n197 = Multiply(x=w445, y=w479) -> (x*y=w444:dbl)
                  n198 = Subtract(x=w479, y=w442) -> (x-y=w468:dbl)
                  "error 2" <- w468
                  n199 = Subtract(x=w479, y=w481) -> (x-y=w461:i32)
                  "dtheta 2" <- w461
                  n200 = Add(x=w444, y="Min Angle2") -> (x+y=→"Current Angle2":dbl)
                  n201 = In Range and Coerce(upper limit=w455, x=w468, lower limit=w451) -> (In Range?=w457:bool)  [unwired: 1 out]
                  n202 = Sign(1:w468) -> (0:w477:dbl)
                  n203 = Divide(x=w461, y=w460) -> (x/y=w459:dbl)
                  "Omega 2" <- w459
                  n204 = case shown="1" w477 {
                    tunnel: [TRUE TRUE FALSE] -> w476
                    tunnel: [TRUE FALSE TRUE] -> w475
                    frame 0, Default {
                    }
                    frame 1 {
                    }
                    frame -1 {
                    }
                  }
                  n205 = case shown="True" w457 {
                    frame False {
                      n206 = local write "Numeric2"(0.0) -> ()
                    }
                    frame True {
                      n207 = local write "Numeric2"(950.0) -> ()
                    }
                  }
                  n208 = Not(x=w457) -> (.not. x?=w467:bool)
                  n209 = call-poly <vilib>:"PID.vi"("output range"=cluster{"output high":dbl, "output low":dbl} {"output high"=0.2, "output low"=-0.2}, "PID gains"="PID gains 4", "process variable"=w459, "setpoint"=-20.0) -> ("output"=w464:dbl)  [unwired: 6 in, 1 out]
                  n210 = And(x=w472, y=w467) -> (x .and. y?=w471:bool)
                  n211 = feedback-in #3(w471) -> ()
                  n212 = And(x=w467, y=w470) -> (x .and. y?=w469:bool)
                  n213 = feedback-in #5(w476) -> ()
                  n214 = feedback-in #6(w475) -> ()
                  n215 = feedback-in #7(w469) -> ()
                  n216 = feedback #8() -> (w380:bool)  [unwired: 1 in]
                  "direction_3b" <- w380
                  n217 = call "SubMotor03.vi"("Reset Counter"=w394, "error in (no error)"=w424, "Duty Cycle"=w368, "A/DIO1 (Pin 13)"=w380, "A/DIO2 (Pin 15)"=w383) -> ("error out"=w421:errorcluster, "Counter Value"=w420:i32)  [unwired: 4 in, 1 out]
                  "Counter Value3" <- w420
                  n218 = Subtract(x=w420, y="Min Encoder3") -> (x-y=w374:dbl)
                  n219 = Subtract(x=w420, y=w395) -> (x-y=w417:dbl)
                  "error3" <- w417
                  n220 = Subtract(x=w420, y=w423) -> (x-y=w411:i32)
                  "dtheta" <- w411
                  n221 = Multiply(x=w373, y=w374) -> (x*y=w372:dbl)
                  n222 = Add(x=w372, y="Min Angle3") -> (x+y=→"Current Angle3":dbl)
                  n223 = In Range and Coerce(upper limit=w407, x=w417, lower limit=w403) -> (In Range?=w393:bool)  [unwired: 1 out]
                  n224 = Sign(1:w417) -> (0:w418:dbl)
                  n225 = Divide(x=w411, y=w410) -> (x/y=w409:dbl)
                  "Omega3 2" <- w409
                  n226 = case shown="True" w393 {
                    frame False {
                      n227 = local write "Numeric3"(0.0) -> ()
                    }
                    frame True {
                      n228 = local write "Numeric3"(950.0) -> ()
                    }
                  }
                  n229 = case shown="0, Default" w418 {
                    tunnel: [TRUE TRUE FALSE] -> w390
                    tunnel: [TRUE FALSE TRUE] -> w391
                    frame 0, Default {
                    }
                    frame 1 {
                    }
                    frame -1 {
                    }
                  }
                  n230 = call-poly <vilib>:"PID.vi"("output range"=cluster{"output high":dbl, "output low":dbl} {"output high"=0.1, "output low"=-0.1}, "PID gains"="PID gains 3", "process variable"=w409, "setpoint"=-23.0) -> ("output"=w414:dbl)  [unwired: 6 in, 1 out]
                  n231 = Not(x=w393) -> (.not. x?=w392:bool)
                  n232 = And(x=w392, y=w390) -> (x .and. y?=w388:bool)
                  n233 = And(x=w392, y=w391) -> (x .and. y?=w389:bool)
                  n234 = Add(x=w414, y=0.6) -> (x+y=w369:dbl)
                  n235 = feedback-in #2(w369) -> ()
                  n236 = case shown="True" TRUE {
                    tunnel: w388 -> [_ w708]
                    tunnel: w389 -> [_ w709]
                    tunnel: [FALSE w709] -> w381
                    tunnel: [FALSE w708] -> w386
                    frame False {
                    }
                    frame True {
                    }
                  }
                  n237 = feedback-in #1(w386) -> ()
                  n238 = feedback-in #8(w381) -> ()
                  n239 = Add(x=w464, y=0.5) -> (x+y=w458:dbl)
                  n240 = feedback-in #4(w458) -> ()
                  n241 = Unbundle(w488) -> (→"Array":dbl[][], →"Array 2":dbl[][], →"Array 3":dbl[][], →"Array 4":dbl[][], →"Array 5":dbl[][], w366:dbl[][])
                  "Array 6" <- w366
                  n242 = call "SubMotor01.vi"("error in (no error)"=w365, "Duty Cycle"=0.4, "A/DIO14 (Pin 32)"=w331, "A/DIO15 (Pin 34)"=w324) -> ("error out"=w364:errorcluster)  [unwired: 5 in, 2 out]
                }
              }
            }
          }
        }
        n243 = local read "stop VI"() -> (w129:bool)
        n244 = Equal?(x=enum32{"train", "run"}."train" ("Tab Control 2"), y=w134) -> (x = y?=w131:bool)
        n245 = Equal?(x=enum32{"control", "train"}."train" ("Tab Control"), y=w132) -> (x = y?=w130:bool)
        n246 = local read "Stop counting"() -> (w124:bool)
        n247 = And(x=w131, y=w130) -> (x .and. y?=w127:bool)
        n248 = Not(x=w129) -> (.not. x?=w128:bool)
        n249 = And(x=w127, y=w128) -> (x .and. y?=w125:bool)
        n250 = Not(x=w124) -> (.not. x?=w126:bool)
        n251 = And(x=w125, y=w126) -> (x .and. y?=w123:bool)
        n252 = case shown="True" w123 {
          frame False {
            w139 = FALSE
            n253 = local write "Vision initialised"(w139) -> ()
            n254 = local write "Encoders initialised"(w139) -> ()
          }
          frame True {
            n255 = local read "stop vision"() -> (w144:bool)
            n256 = Not(x=w144) -> (.not. x?=w143:bool)
            n257 = case shown="True" w143 {
              frame False {
                n258 = local write "Vision initialised"(FALSE) -> ()
              }
              frame True {
                n259 = local read "Tab Control 3"() -> (w148:enum32{"Normal training", "Train using Vision"})
                n260 = Equal?(x=enum32{"Normal training", "Train using Vision"}."Train using Vision" ("Tab Control 3"), y=w148) -> (x = y?=→"Vision initialised":bool)
              }
            }
            n261 = local read "Tab Control 3"() -> (w142:enum32{"Normal training", "Train using Vision"})
            n262 = Equal?(x=enum32{"Normal training", "Train using Vision"}."Normal training" ("Tab Control 3"), y=w142) -> (x = y?=→"Encoders initialised":bool)
          }
        }
      }
      n263 = Build Array(0.0) -> (w31:dbl[])
      n264 = Create Network Stream Writer Endpoint(7:100 ("writer buffer size"), 8:w9, 9:w31, 11:"writer" ("writer name")) -> (0:w23:errorcluster, 3:w8:refnum<k21>)  [unwired: 3 in]
      n265 = while {
        shift-right: [w76] -> w17
        shift-left: w8 -> [w80]
        shift-right: [w74] -> w19
        shift-left: w8 -> [w78]
        shift-right: [w75] -> w18
        shift-left: w23 -> [w79]
        shift-right: [w73] -> w20
        shift-left: w23 -> [w77]
        shift-right: [w72] -> w40
        shift-left: _ -> [w68]
        shift-right: [w71] -> w41
        shift-left: _ -> [w67]
        shift-right: [w70] -> w42
        shift-left: _ -> [w66]
        shift-right: [w69] -> w43
        shift-left: _ -> [w65]
        stop <- w88 stop-if-true
        n266 = Wait (ms)(milliseconds to wait=u32 10) -> ()  [unwired: 1 out]
        n267 = local read "Encoders initialised"() -> (w83:bool)
        n268 = local read "Vision initialised"() -> (w85:bool)
        n269 = And(x="Save", y=w83) -> (x .and. y?=w81:bool)
        n270 = And(x="Save", y=w85) -> (x .and. y?=w82:bool)
        n271 = case shown="True" w82 {
          tunnel: w80 -> [w103 w109]
          tunnel: w79 -> [w102 w108]
          tunnel: [w102 w120] -> w75
          tunnel: [w103 w119] -> w76
          tunnel: [w101 w107] -> w72
          tunnel: [w100 w106] -> w71
          tunnel: [w99 w105] -> w70
          tunnel: [w98 w104] -> w69
          tunnel: w68 -> [w101 _]
          tunnel: w67 -> [w100 _]
          tunnel: w66 -> [w99 _]
          tunnel: w65 -> [w98 _]
          frame False {
          }
          frame True {
            n272 = local read "output cluster 4"() -> (w110:cluster{dbl, dbl})
            n273 = local read "output cluster 3"() -> (w111:cluster{dbl, dbl})
            n274 = local read "output cluster 2"() -> (w116:cluster{dbl, dbl})
            n275 = Cluster To Array(cluster=w110) -> (array=w112:dbl[])
            n276 = Cluster To Array(cluster=w111) -> (array=w114:dbl[])
            n277 = Cluster To Array(cluster=w116) -> (array=w117:dbl[])
            n278 = Build Array(w112) -> (w113:T22)
            n279 = Build Array(w114) -> (w115:T22)
            n280 = Build Array(w117) -> (w118:T22)
            n281 = shared-variable-write(w109, w108, w115) -> (w107:refnum<k21>, w106:errorcluster)  [unwired: 1 in, 1 out]
            n282 = shared-variable-write(w109, w108, w118) -> (w119:refnum<k21>, w120:errorcluster)  [unwired: 1 in, 1 out]
            n283 = shared-variable-write(w109, w108, w113) -> (w105:refnum<k21>, w104:errorcluster)  [unwired: 1 in, 1 out]
          }
        }
        n284 = case shown="True" w81 {
          tunnel: w78 -> [w90 w97]
          tunnel: w77 -> [w89 w96]
          tunnel: [w90 w95] -> w74
          tunnel: [w89 w94] -> w73
          frame False {
          }
          frame True {
            n285 = local read "output cluster"() -> (w93:T6)
            n286 = Cluster To Array(cluster=w93) -> (array=w91:dbl[])
            n287 = Build Array(w91) -> (w92:T22)
            n288 = shared-variable-write(w97, w96, w92) -> (w95:refnum<k21>, w94:errorcluster)  [unwired: 1 in, 1 out]
          }
        }
        n289 = local read "stop VI"() -> (w88:bool)
      }
      n290 = Build Array(0.0) -> (w33:dbl[])
      n291 = Create Network Stream Reader Endpoint(7:100 ("reader buffer size"), 8:w9, 9:w33, 11:"reader" ("reader name")) -> (0:w26:errorcluster, 3:w25:refnum<k21>)  [unwired: 3 in]
      n292 = while {
        tunnel: w25 -> [w63]
        tunnel: w26 -> [w62]
        tunnel: [w61] -> w28
        tunnel: [w60] -> w29
        stop <- w64 stop-if-true
        n293 = shared-variable-read(w63, w62, 6 ("# elements")) -> (w61:refnum<k21>, w60:errorcluster, w57:dbl[][])  [unwired: 1 in, 1 out]
        "data out" <- w57
        n294 = Wait (ms)(milliseconds to wait=u32 100) -> ()  [unwired: 1 out]
        n295 = Index Array(array=w57, index (col) #1=0 ("index (row)"), index (col) #2=1 ("index (col)"), index (col) #3=2 ("index (col)"), index (col) #4=3 ("index (col)"), index (col) #5=4 ("index (row)"), index (col) #6=5 ("index (row)")) -> (element #1=w53:dbl[][], element #2=w52:dbl[][], element #3=w51:dbl[][], element #4=w49:dbl[][], element #5=w46:dbl[][], element #6=w45:dbl[][])  [unwired: 6 in]
        n296 = Bundle(w53, w52, w51, w49, w46, w45) -> (→"output cluster 5":T1)  [unwired: 1 in]
        n297 = local read "stop VI"() -> (w64:bool)
      }
      n298 = Flush Stream(8:w41, 11:w40) -> (0:w35:errorcluster, 3:w34:refnum<k21>)  [unwired: 2 in, 1 out]
      n299 = Flush Stream(8:w18, 11:w17) -> (0:w14:errorcluster, 3:w13:refnum<k21>)  [unwired: 2 in, 1 out]
      n300 = Flush Stream(8:w20, 11:w19) -> (0:w16:errorcluster, 3:w15:refnum<k21>)  [unwired: 2 in, 1 out]
      n301 = Flush Stream(8:w43, 11:w42) -> (0:w37:errorcluster, 3:w36:refnum<k21>)  [unwired: 2 in, 1 out]
      n302 = Destroy Stream Endpoint(8:w35, 11:w34) -> (0:w38:errorcluster)
      n303 = Destroy Stream Endpoint(8:w29, 11:w28) -> (0:w7:errorcluster)
      n304 = Destroy Stream Endpoint(8:w14, 11:w13) -> (0:w21:errorcluster)
      n305 = Destroy Stream Endpoint(8:w16, 11:w15) -> (0:w22:errorcluster)
      n306 = Destroy Stream Endpoint(8:w37, 11:w36) -> (0:w39:errorcluster)
      n307 = Merge Errors(w39, w38, w21, w22, w7) -> (w6:errorcluster)
    }
    frame #2 {
      # "Close"
      n308 = call <vilib>:"Reset myRIO.vi"("error in (no error)"=w799) -> ("error out"=→"error out 2":errorcluster)  [unwired: 10 in]
    }
  }
  n309 = while {
    shift-right: [w811] -> _
    shift-left: _ -> [w816]
    shift-right: [w813] -> _
    shift-left: _ -> [w815]
    shift-right: [w812] -> _
    shift-left: _ -> [w814]
    stop <- w817 stop-if-true
    n310 = local read "Tab Control 3"() -> (w805:enum32{"Normal training", "Train using Vision"})
    n311 = local read "Tab Control"() -> (w808:enum32{"Control", "Train"})
    n312 = Equal?(x=w808, y=enum32{"Control", "Train"}."Control" ("Tab Control")) -> (x = y?=w809:bool)
    n313 = Equal?(x=w805, y=enum32{"Normal training", "Train using Vision"}."Normal training" ("Tab Control 3")) -> (x = y?=w806:bool)
    n314 = Or(x=w809, y=w806) -> (x .or. y?=w810:bool)
    n315 = case shown="True" w810 {
      tunnel: w816 -> [w820 w831]
      tunnel: w815 -> [w819 w830]
      tunnel: w814 -> [w818 w829]
      tunnel: [w819 w828] -> w813
      tunnel: [w818 w827] -> w812
      tunnel: [w820 w826] -> w811
      frame False {
      }
      frame True {
        # "PID control for Motor"
        # "Shoulder Motor control subVI"
        # "Elbow Motor control subVI"
        # "Base Motor control subVI"
        # "PS2 control"
        n316 = local read "Counter Value 3"() -> (w826:i32)
        n317 = local read "Counter Value 2"() -> (w827:i32)
        n318 = xnode "Digital input (1 sample) 6"() -> ("B/DIO3 (Pin 17)"=w918:bool)  [unwired: 1 in, 1 out]
        "B/DIO3 (Pin 17)" <- w918
        n319 = local read "device ID"() -> (w832:refnum<k1>)
        n320 = Tick Count (ms)() -> (millisecond timer value=w828:u32)
        n321 = xnode "Digital input (1 sample) 5"() -> ("B/DIO2 (Pin 15)"=w922:bool)  [unwired: 1 in, 1 out]
        "B/DIO2 (Pin 15)" <- w922
        n322 = Subtract(x="Max Angle 3", y="Min angle 3") -> (x-y=w876:dbl)
        n323 = Subtract(x="Max Encoder Value 3", y="Min Encoder Value 3") -> (x-y=w877:dbl)
        n324 = Subtract(x="Max Angle", y="Min angle") -> (x-y=w849:dbl)
        n325 = Subtract(x="Max Encoder Value", y="Min Encoder Value") -> (x-y=w850:dbl)
        n326 = Subtract(x="Max Angle 2", y="Min angle 2") -> (x-y=w867:dbl)
        n327 = Subtract(x="Max Encoder Value 2", y="Min Encoder Value 2") -> (x-y=w868:dbl)
        n328 = Subtract(x=w826, y=w831) -> (x-y=w883:i32)
        "dtheta3" <- w883
        n329 = Subtract(x=w828, y=w830) -> (x-y=w899:u32)
        "dt" <- w899
        n330 = Subtract(x=w827, y=w829) -> (x-y=w882:i32)
        "dtheta2" <- w882
        n331 = call-poly <vilib>:"Acquire Input Data.vi"("device ID"=w832) -> ("axis info"=→"axis info":T5, "button info"=w835:T4, "direction info"=w836:T3)  [unwired: 14 in, 2 out]
        "button info" <- w835
        "direction info" <- w836
        n332 = xnode "Digital input (1 sample) 4"() -> ("B/DIO4 (Pin 19)"=w823:bool)  [unwired: 1 in, 1 out]
        "B/DIO4 (Pin 19)" <- w823
        n333 = xnode "Digital input (1 sample) 3"() -> ("B/DIO5 (Pin 21)"=w859:bool)  [unwired: 1 in, 1 out]
        "B/DIO5 (Pin 21)" <- w859
        n334 = Divide(x=w876, y=w877) -> (x/y=w878:dbl)
        n335 = Divide(x=w849, y=w850) -> (x/y=w851:dbl)
        n336 = Divide(x=w867, y=w868) -> (x/y=w869:dbl)
        n337 = Not(x=w918) -> (.not. x?=w919:bool)
        n338 = local read "Counter Value 1"() -> (w917:dbl)
        n339 = Or(x="Reset", y=w919) -> (x .or. y?=w920:bool)
        n340 = Multiply(x=w826, y=w878) -> (x*y=w879:dbl)
        n341 = Multiply(x=w827, y=w869) -> (x*y=w870:dbl)
        n342 = Unbundle(w836) -> ("pov 1"=w837:i32)  [unwired: 3 out]
        n343 = Not(x=w922) -> (.not. x?=w923:bool)
        n344 = Not(x=w922) -> (.not. x?=w909:bool)
        n345 = Divide(x=w883, y=w899) -> (x/y=w894:dbl)
        "Omega3" <- w894
        n346 = Divide(x=w882, y=w899) -> (x/y=w825:dbl)
        "Omega2" <- w825
        n347 = Unbundle(w835) -> ("button 1"=w855:bool, "button 2"=w906:bool, "button 3"=w856:bool, "button 4"=w907:bool)  [unwired: 28 out]
        n348 = case shown="-1, Default" w837 {
          tunnel: [FALSE TRUE FALSE] -> w838
          tunnel: [FALSE FALSE TRUE] -> w839
          frame -1, Default {
          }
          frame 90 {
          }
          frame 270 {
          }
        }
        n349 = case shown="-1, Default" w837 {
          tunnel: [FALSE TRUE FALSE] -> w860
          tunnel: [FALSE FALSE TRUE] -> w861
          frame -1, Default {
          }
          frame 180 {
          }
          frame 0 {
          }
        }
        n350 = xnode "Digital input (1 sample) 2"() -> ("B/DIO6 (Pin 23)"=w903:bool)  [unwired: 1 in, 1 out]
        "B/DIO6 (Pin 23)" <- w903
        n351 = Or(x=w920, y=w923) -> (x .or. y?=w921:bool)
        n352 = Or(x="Reset", y=w909) -> (x .or. y?=w908:bool)
        n353 = Add(x=w879, y="Min angle 3") -> (x+y=→"Elbow angle":dbl)
        n354 = Multiply(x=w917, y=w851) -> (x*y=w852:dbl)
        n355 = Add(x=w870, y="Min angle 2") -> (x+y=→"Shoulder angle":dbl)
        n356 = And(x=w855, y=w859) -> (x .and. y?=w858:bool)
        n357 = And(x=w856, y=w823) -> (x .and. y?=w857:bool)
        n358 = And(x=w906, y=w922) -> (x .and. y?=w915:bool)
        n359 = And(x=w907, y=w918) -> (x .and. y?=w916:bool)
        n360 = case shown="True" "Reset" {
          frame False {
          }
          frame True {
            n361 = local read "Max Encoder Value"() -> (w928:dbl)
            n362 = local read "Min Encoder Value"() -> (w927:dbl)
            n363 = Add(x=w928, y=w927) -> (x+y=w926:dbl)
            n364 = Divide(x=w926, y=2.0) -> (x/y=w925:dbl)
            n365 = local write "Counter Value 1"(w925) -> ()
          }
        }
        n366 = case shown="True" w921 {
          frame False {
          }
          frame True {
            n367 = local read "B/DIO3 (Pin 17)"() -> (w932:bool)
            n368 = local read "B/DIO2 (Pin 15)"() -> (w930:bool)
            n369 = Not(x=w932) -> (.not. x?=w931:bool)
            n370 = Not(x=w930) -> (.not. x?=w929:bool)
            n371 = case shown="True" w931 {
              frame False {
              }
              frame True {
                n372 = local read "Min Encoder Value"() -> (w934:dbl)
                n373 = local write "Counter Value 1"(w934) -> ()
              }
            }
            n374 = case shown="True" w929 {
              frame False {
              }
              frame True {
                n375 = local read "Max Encoder Value"() -> (w933:dbl)
                n376 = local write "Counter Value 1"(w933) -> ()
              }
            }
          }
        }
        n377 = xnode "Digital input (1 sample)"() -> ("B/DIO7 (Pin 25)"=w902:bool)  [unwired: 1 in, 1 out]
        "B/DIO7 (Pin 25)" <- w902
        n378 = call-poly <vilib>:"PID.vi"("output range"=cluster{"output high":dbl, "output low":dbl} {"output high"=0.1, "output low"=-0.1}, "PID gains"="PID gains 2", "process variable"=w894, "setpoint"=-23.0) -> ("output"=w892:dbl)  [unwired: 6 in, 1 out]
        n379 = call-poly <vilib>:"PID.vi"("output range"=cluster{"output high":dbl, "output low":dbl} {"output high"=0.2, "output low"=-0.2}, "PID gains"="PID gains", "process variable"=w825, "setpoint"=-20.0) -> ("output"=w886:dbl)  [unwired: 6 in, 1 out]
        n380 = Add(x=w852, y="Min angle") -> (x+y=→"Base angle":dbl)
        n381 = Boolean To (0,1)(Boolean=w915) -> (0, 1=w910:i16)
        n382 = call "SubMotor01.vi"("Frequency [Hz]"=1000.0, "Reset Counter"=w908, "Duty Cycle"=0.4, "A/DIO14 (Pin 32)"=w916, "A/DIO15 (Pin 34)"=w915) -> ()  [unwired: 4 in, 3 out]
        n383 = Boolean To (0,1)(Boolean=w916) -> (0, 1=w913:i16)
        n384 = Not(x=w903) -> (.not. x?=w904:bool)
        n385 = Multiply(x=i16 2, y=w910) -> (x*y=w912:i16)
        n386 = Add(x=w892, y=0.6) -> (x+y=w895:dbl)
        n387 = Add(x=w886, y=0.5) -> (x+y=w888:dbl)
        n388 = Or(x=w904, y="Reset") -> (x .or. y?=w905:bool)
        n389 = Add(x=w912, y=w913) -> (x+y=w914:i16)
        n390 = And(x=w902, y=w861) -> (x .and. y?=w862:bool)
        n391 = And(x=w903, y=w860) -> (x .and. y?=w863:bool)
        n392 = feedback #9() -> (w896:dbl)  [unwired: 1 in]
        n393 = feedback-in #9(w895) -> ()
        n394 = feedback #10() -> (w889:dbl)  [unwired: 1 in]
        n395 = feedback-in #10(w888) -> ()
        n396 = call "SubMotor04.vi"("Frequency [Hz]"=1000.0, "Reset Counter"="Reset", "Duty Cycle"=0.4, "B/DIO15 (Pin 34)"=w839, "B/DIO14 (Pin 32)"=w838) -> ()  [unwired: 4 in, 3 out]
        n397 = case shown="1" w914 {
          frame 0, Default {
          }
          frame 1 {
            n398 = local read "Counter Value 1"() -> (w936:dbl)
            n399 = Increment(x=w936) -> (x+1=w935:dbl)
            n400 = local write "Counter Value 1"(w935) -> ()
          }
          frame 2 {
            n401 = local read "Counter Value 1"() -> (w938:dbl)
            n402 = Decrement(x=w938) -> (x-1=w937:dbl)
            n403 = local write "Counter Value 1"(w937) -> ()
          }
          frame 3 {
          }
        }
        n404 = Not(x=w823) -> (.not. x?=w824:bool)
        n405 = call "SubMotor03.vi"("Frequency [Hz]"=1000.0, "Reset Counter"=w905, "Duty Cycle"=w896, "A/DIO1 (Pin 13)"=w863, "A/DIO2 (Pin 15)"=w862) -> ("Counter Value"=→"Counter Value 3":i32)  [unwired: 4 in, 2 out]
        n406 = Or(x="Reset", y=w824) -> (x .or. y?=w822:bool)
        n407 = call "SubMotor02.vi"("Frequency [Hz]"=1000.0, "Reset Counter"=w822, "Duty Cycle"=w889, "A/DIO4 (Pin 19)"=w858, "A/DIO3 (Pin 17)"=w857) -> ("Counter Value"=→"Counter Value 2":i32)  [unwired: 4 in, 2 out]
        n408 = Wait (ms)(milliseconds to wait=u32 1) -> ()  [unwired: 1 out]
      }
    }
    n409 = local read "Shoulder angle"() -> (w803:dbl)
    n410 = local read "Base angle"() -> (w802:dbl)
    n411 = local read "Elbow angle"() -> (w801:dbl)
    n412 = Bundle("Elbow angle"=w801, "Base angle"=w802, "Shoulder angle"=w803) -> (→"output cluster":T6)  [unwired: 1 in]
    n413 = local read "stop VI"() -> (w817:bool)
  }
